vi "Dpc Get Pin Mask.vi"(0 "hif":u32, 5 "pfsMask":u32, 7 "perc":i32, 9 "ptrid":u16, 11 "error in (no error)":errorcluster) -> (3 "function return":i32, 4 "hif out":u32, 6 "pfsMask out":u32, 8 "perc out":i32, 10 "ptrid out":u16, 15 "error out":errorcluster)   [LabVIEW 2011, in "LVH-Adept.lvlib" / "DPCUTIL.lvlib"]
doc: "DPCAPI BOOL DpcGetPinMask(HANDLE hif, DWORD * pfsMask, ERC * perc, TRID * ptrid);"
uses:
  DPCUTIL.lvlib
  Resources/dpcutil.dll
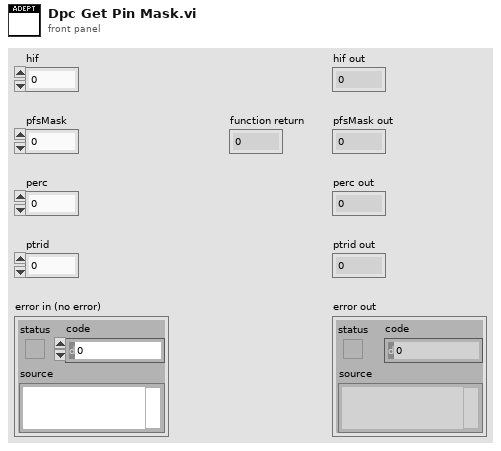
[diagram p1: front panel]
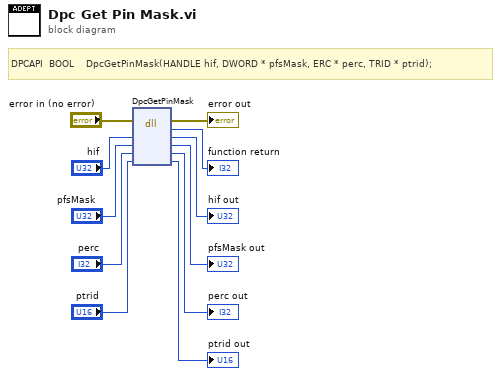
[diagram p0: block diagram]
diagram:
  # "DPCAPI  BOOL    DpcGetPinMask(HANDLE hif, DWORD * pfsMask, ERC * perc, TRID * ptrid);"
  n1 = dll-call lib="C:/github/labviewhacker/LVH-Adept/LabVIEW/vi.lib/LabVIEW Hacker/Adept/Private/Resources/dpcutil.*" fn="DpcGetPinMask"(error in="error in (no error)", "hif"="hif", "pfsMask"="pfsMask", "perc"="perc", "ptrid"="ptrid") -> (error out=→"error out":errorcluster, →"function return":i32, "hif"=→"hif out":u32, "pfsMask"=→"pfsMask out":u32, "perc"=→"perc out":i32, "ptrid"=→"ptrid out":u16)  [unwired: 2 in, 1 out]
